vi "set_laser_onoff.vi"(8 "error in (no error)":errorcluster, 10 "laser on?":bool, 11 "LightSourceAN191011Chameleon in":refnum<class "LightSourceAN191011Chameleon.lvclass">) -> (0 "error out":errorcluster, 3 "LightSourceAN191011Chameleon out":refnum<class "LightSourceAN191011Chameleon.lvclass">)   [LabVIEW 2010, in "LightSourceAN191011Chameleon.lvclass"]
uses:
  LightSourceAN191011Chameleon.lvclass
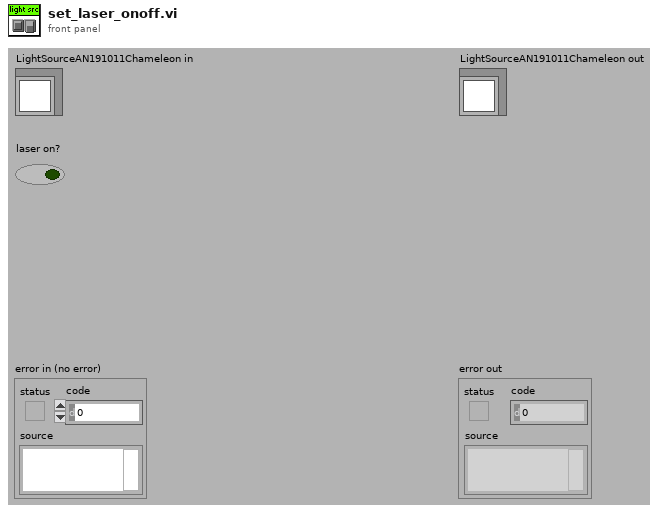
[diagram p1: front panel]
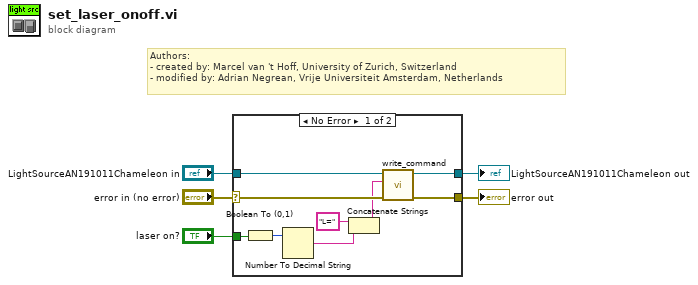
[diagram p0: block diagram]
diagram:
  # "Authors: \n- created by: Marcel van 't Hoff, University of Zurich, Switzerland\n- modified by: Adrian Negrean, Vrije Universiteit Amsterdam, Netherlands"
  n1 = case shown="No Error" "error in (no error)" {
    selector: "error in (no error)" -> [w11 w16]
    tunnel: [w10 w16] -> w4
    tunnel: [w8 w15] -> w2
    tunnel: "LightSourceAN191011Chameleon in" -> [w9 w15]
    tunnel: "laser on?" -> [w6 _]
    frame No Error {
      n2 = Boolean To (0,1)(Boolean=w6) -> (0, 1=w14:i16)
      n3 = Number To Decimal String(number=w14) -> (decimal integer string=w13:string)  [unwired: 1 in]
      n4 = Concatenate Strings("L=" ("string"), w13) -> (w7:string)
      n5 = call-dynamic "write_command.vi"("error in (no error)"=w11, "string to write"=w7, "LightSourceAN191011Chameleon in"=w9) -> ("error out"=w10:errorcluster, "LightSourceAN191011Chameleon out"=w8:refnum<class "LightSourceAN191011Chameleon.lvclass">)  [unwired: 6 in, 1 out]
    }
    frame Error {
    }
  }
  "error out" <- w4
  "LightSourceAN191011Chameleon out" <- w2
